vi "PLC COMM.vi"() -> ()   [LabVIEW 2017]
doc: "Write a Bit array in a DB of a Siemens PLC"
uses:
  <vilib>/DATA AHEAD/SP7/typedefs/PLC Type.ctl
  <vilib>/DATA AHEAD/SP7/functions/write/write single bool.vi
  <vilib>/DATA AHEAD/SP7/functions/read/read bool array.vi
  <vilib>/DATA AHEAD/SP7/functions/read/read Dint array.vi
  Globals/Global manual.vi
  <vilib>/DATA AHEAD/SP7/functions/write/write bool array.vi
  <vilib>/DATA AHEAD/SP7/functions/write/write int array.vi
  <vilib>/DATA AHEAD/SP7/SP7.lvlib
panel:
  out "db 104":T1
  out "DB 103":T2
  out "Manual Operation BD 106":T3
  out "db 104 6.0":bool[](array[boolean])
  out "DB 200":bool[](array[boolean])
  out "Array 2":i32[](array[numeric])
  out "appended array":i32[](array[numeric])
  out "write DB error message 2":string="no error"
  out "write DB 103 data valid.":bool=TRUE
  out "write DB error message":string="no error"
  out "write DB 106 data valid":bool=TRUE
  out "PLC STATUS":bool
  out "db 103 Auto cycle":bool[](array[boolean])
  out "DINT result array":i32[](array[numeric])
  out "auto read BD 104":bool[](array[boolean])
  out "BOOL result array  [byte] 2":bool[](array[boolean])
  out "IP Address":string
  out "AUTOMAODE ON":bool
  out "Alarm DB 105":bool[](array[boolean])
  out "Maintanence Mode On out":bool
  out "Manual DB 106":bool[](array[boolean])
  out "Manual Mode On out":bool
  in  "stop":bool
  in  "timeout [ms]":i32=5000
  in  "error in (no error)":errorcluster
  out "error out":errorcluster
  # "EMG\nCYC START\nPOS 1\nPOS 2\nPOS 3\nPOS 4\nPOS 5\nSERVO HOME\nCYCLE END\nFIXTUR 1\nFIX 2"
  # "SLAVE PART OK\nSLAVE PART NOK\nMAIN PART OK\nMAIN PART NKO\nSCANNER 1OK\nSCANNER 1 NOK\nLASER  OK\nLASER NOK\nSCANNER 2 OK \nSCANNER 2 NOK\nSCANNER 1 ENABLE \nSCANNER1TRIGGER\nSCANNER 2 ENB\nSCANN 2 TRIGG\nLASER ENABLE \nLASER TRIGGER\ncomponent presense\nbleeder presence\nauto manual\nrejection bin\nbleeder ok\nbleeder nok"
  # "bleeder lase neable"
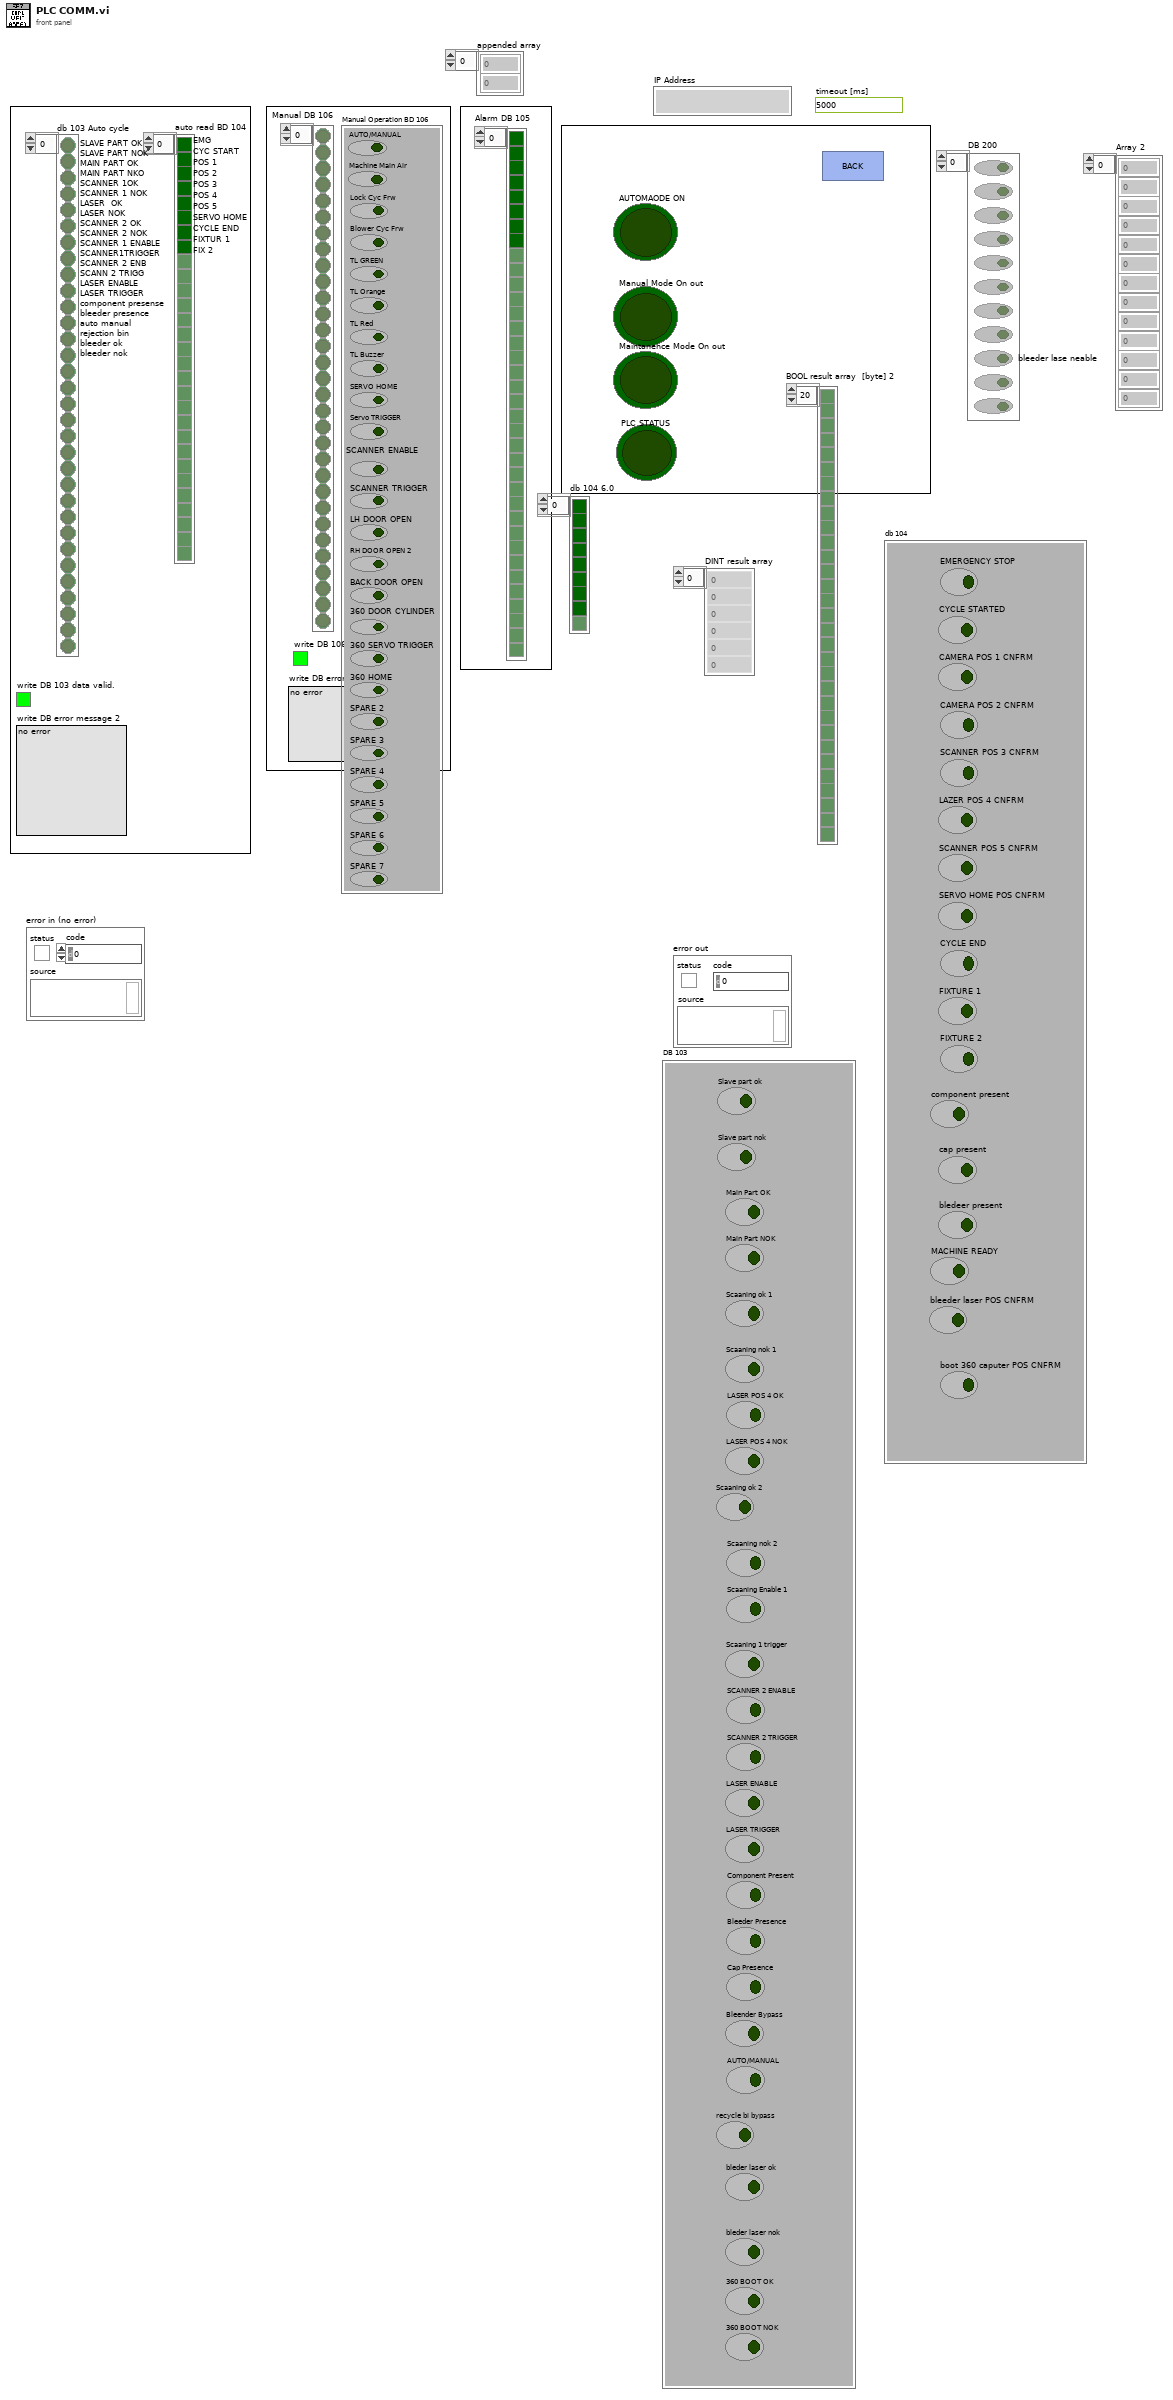
[diagram p1: front panel]
types:
  T1 = cluster{"EMERGENCY STOP":bool, "CYCLE STARTED":bool, "CAMERA POS 1 CNFRM":bool, "CAMERA POS 2 CNFRM":bool, "SCANNER POS 3 CNFRM":bool, "LAZER POS 4 CNFRM":bool, "SCANNER POS 5 CNFRM":bool, "SERVO HOME POS CNFRM":bool, "CYCLE END":bool, "FIXTURE 1":bool, "FIXTURE 2":bool, "component present":bool, "cap present":bool, "bledeer present":bool, "MACHINE READY":bool, "bleeder laser POS CNFRM":bool, "boot 360 caputer POS CNFRM":bool}
  T2 = cluster{"Slave part ok":bool, "Slave part nok":bool, "Main Part OK":bool, "Main Part NOK":bool, "Scaaning ok 1":bool, "Scaaning nok 1":bool, "LASER POS 4 OK":bool, "LASER POS 4 NOK":bool, "Scaaning ok 2":bool, "Scaaning nok 2":bool, "Scaaning Enable 1":bool, "Scaaning 1 trigger":bool, "SCANNER 2 ENABLE":bool, "SCANNER 2 TRIGGER":bool, "LASER ENABLE":bool, "LASER TRIGGER":bool, "Component Present":bool, "Bleeder Presence":bool, "Cap Presence":bool, "Bleender Bypass":bool, "AUTO/MANUAL":bool, "recycle bi bypass":bool, "bleder laser ok":bool, "bleder laser nok":bool, "360 BOOT OK":bool, "360 BOOT NOK":bool}
  T3 = cluster{"AUTO/MANUAL":bool, "Machine Main Air":bool, "Lock Cyc Frw":bool, "Blower Cyc Frw":bool, "TL GREEN":bool, "TL Orange":bool, "TL Red":bool, "TL Buzzer":bool, "SERVO HOME":bool, "Servo TRIGGER":bool, "SCANNER ENABLE":bool, "SCANNER TRIGGER":bool, "LH DOOR OPEN":bool, "RH DOOR OPEN 2":bool, "BACK DOOR OPEN":bool, "360 DOOR CYLINDER":bool, "360 SERVO TRIGGER":bool, "360 HOME":bool, "SPARE 2":bool, "SPARE 3":bool, "SPARE 4":bool, "SPARE 5":bool, "SPARE 6":bool, "SPARE 7":bool}
  T4 = typedef "SP7.lvlib/PLC Type.ctl" = enum16{"S7 200", "S7 300/400", "S7 1200", "S7 1500", "LOGO!8"}
  T5 = typedef "IMAQdx.ctl" = refnum<k21>
  T6 = cluster{"Scanner Com Port":refnum<visa-resource-name>, "Printer Com Port":refnum<visa-resource-name>, "Printer Baud rate":u32, "Printer Serial type":enum16{"RTU", "ASCII"}, "Printer Parity":u16, "Scanner Serial type":enum16{"RTU", "ASCII"}, "Scanner Parity":u16, "Scanner Baud rate":u32, "IP Address":string, "port":u16, "Camare S.V. Selection":T5, "Camare T.V. Selection":T5, "recycle bin Bypass":bool, "Camare 360 BOOT Selection":T5}
  T7 = typedef "SP7.lvlib/S7 Connection.ctl" = cluster{"TCP Connection Ref":refnum<k5>, "IP address":string, "timeout ms":i32, "Connected?":bool, "PLC Type":T4, "Rack S7 400":u8, "Slot S7 400":u8, "PDU Size":u16, "connection semaphore":T8}
  T8 = typedef "Semaphore RefNum" = refnum<k1>
  T9 = cluster{"360 CYCLE START":bool, "360 cycle time":dbl}
  T10 = cluster{"BOOL result array  [byte][0]":bool, "BOOL result array  [byte][1]":bool, "BOOL result array  [byte][2]":bool, "BOOL result array  [byte][3]":bool, "BOOL result array  [byte][4]":bool, "BOOL result array  [byte][5]":bool, "BOOL result array  [byte][6]":bool, "BOOL result array  [byte][7]":bool, "BOOL result array  [byte][8]":bool, "BOOL result array  [byte][9]":bool, "BOOL result array  [byte][10]":bool, "BOOL result array  [byte][11]":bool, "BOOL result array  [byte][12]":bool, "BOOL result array  [byte][13]":bool, "BOOL result array  [byte][14]":bool, "BOOL result array  [byte][15]":bool, "BOOL result array  [byte][16]":bool}
  T11 = cluster{"BOOL result array  [byte][0]":bool, "BOOL result array  [byte][1]":bool, "BOOL result array  [byte][2]":bool, "BOOL result array  [byte][3]":bool, "BOOL result array  [byte][4]":bool, "BOOL result array  [byte][5]":bool, "BOOL result array  [byte][6]":bool, "BOOL result array  [byte][7]":bool, "BOOL result array  [byte][8]":bool, "BOOL result array  [byte][9]":bool, "BOOL result array  [byte][10]":bool, "BOOL result array  [byte][11]":bool, "BOOL result array  [byte][12]":bool, "BOOL result array  [byte][13]":bool, "BOOL result array  [byte][14]":bool, "BOOL result array  [byte][15]":bool, "BOOL result array  [byte][16]":bool, "BOOL result array  [byte][17]":bool, "BOOL result array  [byte][18]":bool, "BOOL result array  [byte][19]":bool, "BOOL result array  [byte][20]":bool, "BOOL result array  [byte][21]":bool, "BOOL result array  [byte][22]":bool, "BOOL result array  [byte][23]":bool, "BOOL result array  [byte][24]":bool, "BOOL result array  [byte][25]":bool, "BOOL result array  [byte][26]":bool, "BOOL result array  [byte][27]":bool, "BOOL result array  [byte][28]":bool, "BOOL result array  [byte][29]":bool, "BOOL result array  [byte][30]":bool, "BOOL result array  [byte][31]":bool, "BOOL result array  [byte][32]":bool, "BOOL result array  [byte][33]":bool, "BOOL result array  [byte][34]":bool, "BOOL result array  [byte][35]":bool, "BOOL result array  [byte][36]":bool, "BOOL result array  [byte][37]":bool, "BOOL result array  [byte][38]":bool, "BOOL result array  [byte][39]":bool, "BOOL result array  [byte][40]":bool, "BOOL result array  [byte][41]":bool, "BOOL result array  [byte][42]":bool, "BOOL result array  [byte][43]":bool, "BOOL result array  [byte][44]":bool, "BOOL result array  [byte][45]":bool, "BOOL result array  [byte][46]":bool, "BOOL result array  [byte][47]":bool, "BOOL result array  [byte][48]":bool, "BOOL result array  [byte][49]":bool, "BOOL result array  [byte][50]":bool, "BOOL result array  [byte][51]":bool, "BOOL result array  [byte][52]":bool, "BOOL result array  [byte][53]":bool, "BOOL result array  [byte][54]":bool, "BOOL result array  [byte][55]":bool}
  T12 = cluster{"BOOL result array  [byte][0]":bool, "BOOL result array  [byte][1]":bool, "BOOL result array  [byte][2]":bool, "BOOL result array  [byte][3]":bool, "BOOL result array  [byte][4]":bool, "BOOL result array  [byte][5]":bool, "BOOL result array  [byte][6]":bool, "BOOL result array  [byte][7]":bool, "BOOL result array  [byte][8]":bool, "BOOL result array  [byte][9]":bool, "BOOL result array  [byte][10]":bool, "BOOL result array  [byte][11]":bool, "BOOL result array  [byte][12]":bool, "BOOL result array  [byte][13]":bool, "BOOL result array  [byte][14]":bool, "BOOL result array  [byte][15]":bool, "BOOL result array  [byte][16]":bool, "BOOL result array  [byte][17]":bool, "BOOL result array  [byte][18]":bool, "BOOL result array  [byte][19]":bool, "BOOL result array  [byte][20]":bool, "BOOL result array  [byte][21]":bool, "BOOL result array  [byte][22]":bool, "BOOL result array  [byte][23]":bool, "BOOL result array  [byte][24]":bool, "BOOL result array  [byte][25]":bool, "BOOL result array  [byte][26]":bool, "BOOL result array  [byte][27]":bool, "BOOL result array  [byte][28]":bool, "BOOL result array  [byte][29]":bool, "BOOL result array  [byte][30]":bool, "BOOL result array  [byte][31]":bool, "BOOL result array  [byte][32]":bool, "BOOL result array  [byte][33]":bool, "BOOL result array  [byte][34]":bool, "BOOL result array  [byte][35]":bool, "BOOL result array  [byte][36]":bool, "BOOL result array  [byte][37]":bool, "BOOL result array  [byte][38]":bool, "BOOL result array  [byte][39]":bool, "BOOL result array  [byte][40]":bool, "BOOL result array  [byte][41]":bool}
  T13 = enum32{"invalid app kind", "Development System", "Run Time System", "Student Edition", "Embedded LabVIEW", "Evaluation", "Custom"}
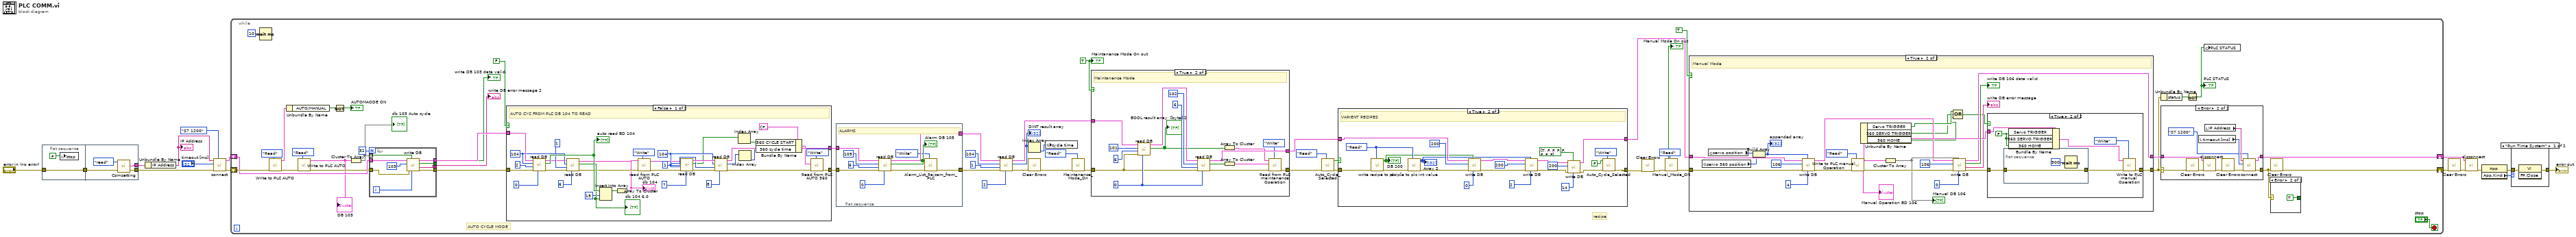
[diagram p0: block diagram]
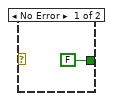
[diagram p5: hidden frame]
diagram:
  n1 = flat-sequence {
    tunnel: "error in (no error)" -> [w18]
    tunnel: [w18] -> w4
    tunnel: [w20] -> w5
    tunnel: w4 -> [w21]
    tunnel: [w19] -> w3
    frame #0 {
      n2 = local write "stop"(FALSE) -> ()
    }
    frame #1 {
      n3 = call "Comsetting.vi"("error in"=w21, "Enum"=enum16{"read", "write"}."read") -> ("error our"=w20:errorcluster, "Cluster Out"=w19:T6)  [unwired: 1 in, 1 out]
    }
  }
  n4 = Unbundle By Name(w3) -> ("IP Address"=w1:string)
  "IP Address" <- w1
  n5 = call <vilib>:"connect.vi"("PLC Type"=PLC_Type."S7 1200" ("PLC Type 2"), "error in (no error)"=w5, "timeout [ms]"="timeout [ms]", "IP address"=w1) -> ("error out"=w15:errorcluster, "S7 Connection out"=w14:T7)  [unwired: 6 in]
  n6 = while {
    shift-right: [w23] -> w8
    shift-left: w15 -> [w46]
    shift-right: [w75] -> w13
    shift-left: w14 -> [w44]
    stop <- "stop" stop-if-true
    w57 = TRUE
    # "recipe"
    # "AUTO CYCLE MODE"
    n7 = Wait (ms)(milliseconds to wait=u32 10) -> ()  [unwired: 1 out]
    n8 = call "Write to PLC AUTO.vi"("Enum"=enum16{"Write", "Read"}."Read", "error in (no error)"=w46) -> ("error in (no error) 2"=w64:errorcluster, "In 2"=w62:T2)  [unwired: 8 in]
    n9 = Unbundle By Name(w62) -> ("AUTO/MANUAL"=w48:bool)
    n10 = call "Write to PLC AUTO.vi"("Enum"=enum16{"Write", "Read"}."Read", "error in (no error)"=w64) -> ("error in (no error) 2"=w43:errorcluster, "In 2"=w26:T2)  [unwired: 8 in]
    "DB 103" <- w26
    n11 = Not(x=w48) -> (.not. x?=→"AUTOMAODE ON":bool)
    n12 = Cluster To Array(cluster=w26) -> (array=w27:bool[])
    "db 103 Auto cycle" <- w27
    n13 = for {
      N: 32 -> [_]
      tunnel: [w81] -> w41
      tunnel: [w80] -> w40
      tunnel: w27 -> [w78] mode=indexing
      tunnel: w44 -> [w84]
      tunnel: [w82] -> w42
      tunnel: w43 -> [w83]
      tunnel: [w77] -> w24
      i -> [w76]
      n14 = call-poly <vilib>:"write DB.vi"("Item offset [bit]"=w76, "BOOL"=w78, "error in (no error)"=w83, "Data Block #"=u16 103, "S7 Connection in"=w84) -> ("error out"=w77:errorcluster, "write DB error message"=w80:string, "write DB data valid?"=w81:bool, "S7 Connection out"=w82:T7)  [unwired: 3 in]
    }
    "write DB 103 data valid." <- w41
    "write DB error message 2" <- w40
    n15 = case shown="False" FALSE {
      tunnel: [w174 w204] -> w61
      tunnel: [w178 w205] -> w60
      tunnel: w24 -> [w200 w204]
      tunnel: w42 -> [w199 w205]
      frame False {
        w182 = u16 1 ("Items # [byte]")
        w185 = u16 104 ("Data Block #")
        w195 = u16 104 ("Data Block #")
        # "AUTO CYC FROM PLC DB 104 TO READ"
        n16 = call-poly <vilib>:"read DB.vi"("Item offset [byte]"=u32 0, "error in (no error)"=w200, "Items # [byte]"=u16 2, "Data Block #"=w195, "S7 Connection in"=w199) -> ("error out"=w196:errorcluster, "BOOL result array  [byte]"=w198:bool[], "S7 Connection out"=w193:T7)  [unwired: 4 in]
        "auto read BD 104" <- w198
        n17 = call-poly <vilib>:"read DB.vi"("Item offset [byte]"=u32 6, "error in (no error)"=w196, "Items # [byte]"=u16 1, "Data Block #"=w195, "S7 Connection in"=w193) -> ("error out"=w191:errorcluster, "BOOL result array  [byte]"=w192:bool[], "S7 Connection out"=w179:T7)  [unwired: 4 in]
        "db 104 6.0" <- w192
        n18 = Insert Into Array(array=w198, index=15, new element=w192) -> (w197:bool[])
        n19 = Array To Cluster(array=w197) -> (cluster=w188:T10)
        "db 104" <- w188
        n20 = call "read from PLC AUTO.vi"("Enum"=enum16{"Write", "Read"}."Write", "error in (no error)"=w191, "In"=w188) -> ("error in (no error) 2"=w181:errorcluster)  [unwired: 7 in, 1 out]
        n21 = call-poly <vilib>:"read DB.vi"("Item offset [byte]"=u32 7, "error in (no error)"=w181, "Items # [byte]"=w182, "Data Block #"=w185, "S7 Connection in"=w179) -> ("error out"=w183:errorcluster, "BOOL result array  [byte]"=w177:bool[], "S7 Connection out"=w186:T7)  [unwired: 4 in]
        n22 = call-poly <vilib>:"read DB.vi"("Item offset [byte]"=u32 8, "error in (no error)"=w183, "items #"=w182, "Data Block #"=w185, "S7 Connection in"=w186) -> ("error out"=w175:errorcluster, "DINT result array"=w180:i32[], "S7 Connection out"=w178:T7)  [unwired: 4 in]
        n23 = Index Array(array=w177) -> (element=w172:bool)  [unwired: 1 in]
        n24 = Index Array(array=w180) -> (element=w171:i32)  [unwired: 1 in]
        n25 = Bundle By Name(cluster=T9 {"360 CYCLE START"=FALSE, "360 cycle time"=0.0} ("IN"), "360 CYCLE START"=w172, "360 cycle time"=w171) -> (w170:T9)
        n26 = call "Read from PLC AUTO 360.vi"("Enum"=enum16{"Write", "Read"}."Write", "error in (no error)"=w175, "IN"=w170) -> ("error in (no error) 2"=w174:errorcluster)  [unwired: 7 in, 1 out]
      }
      frame True {
      }
    }
    n27 = flat-sequence {
      tunnel: [w119] -> w54
      tunnel: [w118] -> w52
      tunnel: w60 -> [w111]
      tunnel: w61 -> [w110]
      frame #0 {
        # "ALARMS"
        n28 = call-poly <vilib>:"read DB.vi"("Item offset [byte]"=u32 0, "error in (no error)"=w110, "Items # [byte]"=u16 6, "Data Block #"=u16 105, "S7 Connection in"=w111) -> ("error out"=w114:errorcluster, "BOOL result array  [byte]"=w113:bool[], "S7 Connection out"=w118:T7)  [unwired: 4 in]
        "Alarm DB 105" <- w113
        n29 = call "Alarm_List_Raicam_from_PLC.vi"("Enum"=enum16{"Write", "Read"}."Write", "error in (no error)"=w114, "Alarm In"=w113) -> ("error in (no error) 2"=w119:errorcluster)  [unwired: 7 in, 1 out]
      }
    }
    n30 = call-poly <vilib>:"read DB.vi"("Item offset [byte]"=u32 2, "error in (no error)"=w54, "items #"=u16 1, "Data Block #"=u16 104, "S7 Connection in"=w52) -> ("error out"=w55:errorcluster, "DINT result array"=w31:i32[], "S7 Connection out"=w53:T7)  [unwired: 4 in]
    "DINT result array" <- w31
    n31 = Index Array(array=w31) -> (element=w32:i32)  [unwired: 1 in]
    n32 = call <vilib>:"Clear Errors.vi"("error in (no error)"=w55) -> ("error out"=w66:errorcluster)  [unwired: 5 in, 1 out]
    n33 = global write "Global manual.vi" "cycle time"(w32) -> ()
    n34 = call "Maintanence_Mode_On.vi"("Enum"=enum16{"Write", "Read"}."Read", "Error In"=w66) -> ("Error Out"=w68:errorcluster)  [unwired: 8 in, 1 out]
    n35 = case shown="True" w57 {
      tunnel: w68 -> [w206 w216]
      tunnel: w53 -> [w207 w221]
      tunnel: [w206 w214] -> w39
      tunnel: [w207 w223] -> w34
      frame False {
      }
      frame True {
        w218 = u32 0 ("Item offset [byte]")
        # "Maintanence Mode"
        n36 = call-poly <vilib>:"read DB.vi"("Item offset [byte]"=w218, "error in (no error)"=w216, "Items # [byte]"=u16 6, "Data Block #"=u16 101, "S7 Connection in"=w221) -> ("BOOL result array  [byte]"=w208:bool[], "S7 Connection out"=w220:T7)  [unwired: 4 in, 1 out]
        "BOOL result array  [byte] 2" <- w208
        n37 = call-poly <vilib>:"read DB.vi"("Item offset [byte]"=w218, "error in (no error)"=w216, "Items # [byte]"=u16 6, "Data Block #"=u16 102, "S7 Connection in"=w220) -> ("error out"=w215:errorcluster, "BOOL result array  [byte]"=w212:bool[], "S7 Connection out"=w223:T7)  [unwired: 4 in]
        n38 = Array To Cluster(array=w208) -> (cluster=w213:T11)
        n39 = Array To Cluster(array=w212) -> (cluster=w211:T12)
        n40 = call "Read from PLC maintanence Operation.vi"("Enum"=enum16{"Write", "Read"}."Write", "error in (no error)"=w215, "OUT plc"=w211, "input plc Input in"=w213) -> ("error in (no error) 2"=w214:errorcluster)  [unwired: 3 in, 2 out]
      }
    }
    n41 = call "Auto_Cycle_Selected.vi"("Enum"=enum16{"Write", "Read"}."Read", "Error In"=w39) -> ("Error Out"=w37:errorcluster, "Manual Mode On out"=w35:bool)  [unwired: 8 in]
    n42 = case shown="True" w35 {
      tunnel: [w86 w96] -> w36
      tunnel: w37 -> [w86 w107]
      tunnel: w34 -> [w85 w103]
      tunnel: [w85 w89] -> w33
      frame False {
      }
      frame True {
        w108 = enum16{"Write", "Read"}."Read" ("Enum")
        # "VARIENT RECIPES"
        n43 = call "write recipe to plc.vi"("Enum"=w108, "Error In"=w107) -> ("Error Out"=w109:errorcluster, "Array 2"=w102:bool[])  [unwired: 8 in]
        "DB 200" <- w102
        n44 = call "recip[e to plc int value.vi"("Enum"=w108, "Error In"=w109) -> ("Error Out"=w104:errorcluster, "Array 2"=w94:i32[])  [unwired: 8 in]
        "Array 2" <- w94
        n45 = call-poly <vilib>:"write DB.vi"("Item offset [byte]"=u32 0, "BOOL input array [byte]"=w102, "error in (no error)"=w104, "Data Block #"=u16 200, "S7 Connection in"=w103) -> ("error out"=w98:errorcluster, "S7 Connection out"=w100:T7)  [unwired: 3 in, 2 out]
        n46 = call-poly <vilib>:"write DB.vi"("Item offset [byte]"=u32 2, "INT input array"=w94, "error in (no error)"=w98, "Data Block #"=u16 200, "S7 Connection in"=w100) -> ("error out"=w92:errorcluster, "S7 Connection out"=w90:T7)  [unwired: 3 in, 2 out]
        n47 = call-poly <vilib>:"write DB.vi"("Item offset [byte]"=u32 14, "BOOL input array [byte]"=bool[] [TRUE, FALSE, FALSE, FALSE, FALSE, FALSE, FALSE, FALSE], "error in (no error)"=w92, "Data Block #"=u16 200, "S7 Connection in"=w90) -> ("error out"=w91:errorcluster, "S7 Connection out"=w89:T7)  [unwired: 3 in, 2 out]
        n48 = call "Auto_Cycle_Selected.vi"("Enum"=enum16{"Write", "Read"}."Write", "Error In"=w91, "Manual mode on in"=FALSE) -> ("Error Out"=w96:errorcluster)  [unwired: 7 in, 1 out]
      }
    }
    n49 = call <vilib>:"Clear Errors.vi"("error in (no error)"=w36) -> ("error out"=w69:errorcluster)  [unwired: 5 in, 1 out]
    n50 = call "Manual_Mode_ON.vi"("Enum"=enum16{"Write", "Read"}."Read", "Error In"=w69) -> ("Error Out"=w71:errorcluster, "Manual Mode On out"=→"Manual Mode On out":bool)  [unwired: 8 in]
    n51 = case shown="True" TRUE {
      tunnel: w71 -> [w120 w130]
      tunnel: w33 -> [w121 w129]
      tunnel: [w120 w136] -> w28
      tunnel: [w121 w135] -> w73
      frame False {
      }
      frame True {
        # "Manual Mode"
        n52 = global read "Global manual.vi" "servo 360 position"() -> (w127:i16)
        n53 = global read "Global manual.vi" "servo position"() -> (w134:i16)
        n54 = Build Array(w134, w127) -> (w133:i16[])
        "appended array" <- w133
        n55 = call-poly <vilib>:"write DB.vi"("Item offset [byte]"=u32 4, "INT input array"=w133, "error in (no error)"=w130, "Data Block #"=u16 106, "S7 Connection in"=w129) -> ("error out"=w126:errorcluster, "S7 Connection out"=w128:T7)  [unwired: 3 in, 2 out]
        n56 = call "Write to PLC manual Operation.vi"("Enum"=enum16{"Write", "Read"}."Read", "Error In"=w126) -> ("Error Out"=w142:errorcluster, "Manual Operation In 2"=w138:T3)  [unwired: 8 in]
        "Manual Operation BD 106" <- w138
        n57 = Unbundle By Name(w138) -> ("Servo TRIGGER"=w125:bool, "360 SERVO TRIGGER"=w124:bool, "360 HOME"=w122:bool)
        n58 = Cluster To Array(cluster=w138) -> (array=w141:bool[])
        "Manual DB 106" <- w141
        n59 = Compound Arithmetic op=OR(w125, w124, w122) -> (w123:bool)
        n60 = call-poly <vilib>:"write DB.vi"("Item offset [byte]"=u32 0, "BOOL input array [byte]"=w141, "error in (no error)"=w142, "Data Block #"=u16 106, "S7 Connection in"=w128) -> ("error out"=w139:errorcluster, "write DB error message"=→"write DB error message":string, "write DB data valid?"=→"write DB 106 data valid":bool, "S7 Connection out"=w135:T7)  [unwired: 3 in]
        n61 = case shown="True" w123 {
          tunnel: w139 -> [w146 w149]
          tunnel: [w146 w152] -> w136
          tunnel: w138 -> [_ w151]
          frame False {
          }
          frame True {
            w147 = FALSE
            n62 = flat-sequence {
              tunnel: [w155] -> w148
              tunnel: w149 -> [w155]
              frame #0 {
                n63 = Wait (ms)(milliseconds to wait=u32 500) -> ()  [unwired: 1 out]
              }
            }
            n64 = Bundle By Name(cluster=w151, "Servo TRIGGER"=w147, "360 SERVO TRIGGER"=w147, "360 HOME"=w147) -> (w150:T3)
            n65 = call "Write to PLC manual Operation.vi"("Enum"=enum16{"Write", "Read"}."Write", "Error In"=w148, "Manual Operation In"=w150) -> ("Error Out"=w152:errorcluster)  [unwired: 7 in, 1 out]
          }
        }
      }
    }
    n66 = Unbundle By Name(w28) -> ("status"=w30:bool)
    n67 = case shown="Error" w28 {
      selector: w28 -> [w159 w168]
      tunnel: [w158 w165] -> w75
      tunnel: [w159 w166] -> w74
      tunnel: w73 -> [w158 w161]
      frame No Error {
      }
      frame Error {
        n68 = call <vilib>:"Clear Errors.vi"("error in (no error)"=w168) -> ("error out"=w169:errorcluster)  [unwired: 5 in, 1 out]
        n69 = local read "timeout [ms]"() -> (w163:i32)
        n70 = call <vilib>:"disconnect.vi"("error in (no error)"=w169, "S7 Connection in"=w161) -> ("error out"=w167:errorcluster)  [unwired: 8 in, 1 out]
        n71 = local read "IP Address"() -> (w164:string)
        n72 = call <vilib>:"Clear Errors.vi"("error in (no error)"=w167) -> ("error out"=w162:errorcluster)  [unwired: 5 in, 1 out]
        n73 = call <vilib>:"connect.vi"("PLC Type"=PLC_Type."S7 1200" ("PLC Type 2"), "error in (no error)"=w162, "timeout [ms]"=w163, "IP address"=w164) -> ("error out"=w166:errorcluster, "S7 Connection out"=w165:T7)  [unwired: 6 in]
      }
    }
    n74 = Not(x=w30) -> (.not. x?=w29:bool)
    "PLC STATUS" <- w29
    n75 = global write "Global manual.vi" "PLC STATUS"(w29) -> ()
    n76 = call <vilib>:"Clear Errors.vi"("error in (no error)"=w74) -> ("error out"=w23:errorcluster)  [unwired: 5 in, 1 out]
    n77 = case shown="Error" w74 {
      tunnel: [FALSE ("IN") TRUE ("IN")] -> _
      frame No Error {
      }
      frame Error {
      }
    }
    "Maintanence Mode On out" <- w57
  }
  n78 = call <vilib>:"Clear Errors.vi"("error in (no error)"=w8) -> ("error out"=w7:errorcluster)  [unwired: 5 in, 1 out]
  n79 = call <vilib>:"disconnect.vi"("error in (no error)"=w7, "S7 Connection in"=w13) -> ("error out"=w9:errorcluster)  [unwired: 8 in, 1 out]
  n80 = property class="App"(error in=w9) -> (error out=w11:errorcluster, "App.Kind"=w12:T13)  [unwired: 1 in, 1 out]
  n81 = case shown="\"Run Time System\"" w12 {
    tunnel: w11 -> [w225 w226]
    tunnel: [w224 w226] -> w10
    frame "Run Time System" {
      n82 = invoke class="VI" method="FP.Close"(error in=w225) -> (error out=w224:errorcluster)  [unwired: 2 in, 2 out]
    }
    frame "Student Edition", Default {
    }
  }
  "error out" <- w10
